vi "_ShowMessage.vi"(1 "TwoButton? (F)":bool, 2 "Message":string) -> (0 "Ok?":bool)   [LabVIEW 2015]
uses:
  Type/_RT Command.ctl
panel:
  out "quit":bool
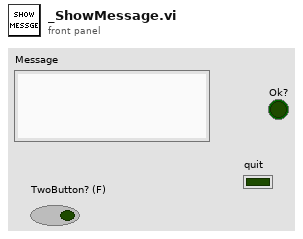
[diagram p1: front panel]
types:
  T1 = typedef "_RT Command.ctl" = enum16{"Start", "Stop", "Runtime Update", "Get Data", "Get Info", "Get Status", "Get Param", "Get Config", "Get Table", "Read ADC", "Set Oscillator", "Update Config", "Update Table", "Set All Pol", "Set Pol and DC", "Set Max Mass", "Toggle RP", "Toggle EL", "Set PIC", "Initialize Turbo", "Send Turbo Comm", "Close Turbo", "P1", "P2", "P3", "Send Serial", "Set LC Out", "Get LC In", "Read VAC", "Test Table", "Toggle Power", "Get Startup", "Set Startup", "Get ADC Table", "Set ADC Table", "Get Brief Status", "Get Detail Status", "Auxiliary Update", "Set CC Logics", "Set CC Input Logics", "Ignore Error"}
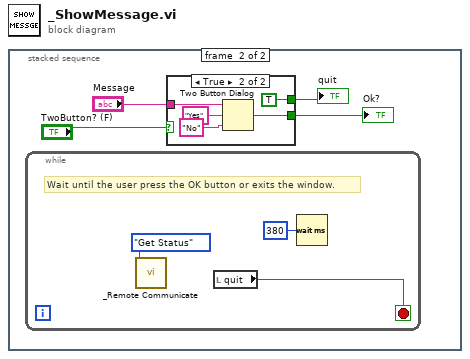
[diagram p0: block diagram]
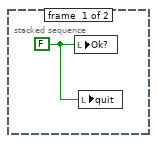
[diagram p2: hidden frame]
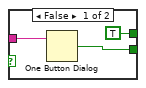
[diagram p3: hidden frame]
diagram:
  n1 = stacked-sequence {
    frame #0 {
      w1 = FALSE ("Ok?")
      n2 = local write "Ok?"(w1) -> ()
      n3 = local write "quit"(w1) -> ()
    }
    frame #1 {
      n4 = while {
        stop <- w14 stop-if-true
        # "Wait until the user press the OK button or exits the window."
        n5 = call "_Remote Communicate.vi"("Command"=_RT_Command."Get Status") -> ()  [unwired: 5 in, 4 out]
        n6 = local read "quit"() -> (w14:bool)
        n7 = Wait (ms)(milliseconds to wait=u32 380) -> ()  [unwired: 1 out]
      }
      n8 = case shown="True" "TwoButton? (F)" {
        tunnel: "Message" -> [w8 w13]
        tunnel: [w7 w12] -> w4
        tunnel: [TRUE TRUE] -> w2
        frame False {
          n9 = One Button Dialog(message=w8) -> (true=w7:bool)  [unwired: 1 in]
        }
        frame True {
          n10 = Two Button Dialog(message=w13, 1:"No" ("F button name (\"Cancel\")"), 2:"Yes" ("T button name (\"OK\")")) -> (T button?=w12:bool)
        }
      }
      "Ok?" <- w4
      "quit" <- w2
    }
  }
